vi "Analyse Doppler waveforms.vi"() -> ()   [LabVIEW 2022 SP3]
uses:
  Instance           1 33Saved   Analyse Doppler waveforms .vi
  Instance           6 33Saved   Analyse Doppler waveforms .vi
  Instance           5 33Saved   Analyse Doppler waveforms .vi
  Instance           2 33Saved   Analyse Doppler waveforms .vi
  <vilib>/express/express analysis/Spectral/Block/exnSpectralBlock spectral measurements power poly.vi
  <vilib>/express/express analysis/Spectral/Block/exnSpectralBlock spectral measurements power DDT.vi
  Instance           7 33Saved   Analyse Doppler waveforms .vi
  Instance           8 33Saved   Analyse Doppler waveforms .vi
  <vilib>/express/express analysis/Spectral/XNode/ExpressSpectralMeasurementsBlockNode.xnode
  <vilib>/gmath/NI_Gmath.lvlib
panel:
  out "Number of samples 2":dbl
  out "Waveform Graph 4":dbl[](graph)
  out "Array 3":dbl[](array[numeric])
  out "Array 2":i32[](array[numeric])
  out "cursor y  index":dbl
  out "cursor x  index":dbl
  out "Spectrogram":dbl[][](graph)
  out "Number of samples":i32
  in  "Frame time shift":i32(slide)=290 caption="in mumber of samples" min=4 max=512 step=2 scale=0.0..512.0
  out "Sampling frequency":dbl
  in  "window selector":i32(ring)=4 items=["Rectangular", "Blackman", "Hamming", "Hanning", "Gaussian"]
  out "Waveform Graph 3":dynamicdata(graph)=[{"t0"=timestamp(0 s since 1904-01-01), "dt"=31.372549019607842, "Y"=array[255 elements], "attributes"=variant("NI_ChannelName"=variant(string "Dev1/ai0 (Power Spectrum)"), "NI_ExpIsRelativeTime"=variant(bool TRUE), "NI_ExpStartTimeStamp"=variant(timestamp timestamp(3271175312.342312 s since 1904-01-01)), "NI_ExpTimeStamp"=variant(timestamp timestamp(3271175312.8210626 s since 1904-01-01)), "NI_ExpXDimension"=variant(string "f"), "NI_OriginalChannelName"=variant(string "Dev1/ai0"))}]
  in  "Frame width":i32(slide)=342 min=2 max=1024 step=2 scale=0.0..1024.0
  in  "stop":bool
  in  "Begin Sample":i32(slide)=2401 min=1 max=50000 step=10 scale=0.0..50000.0
  out "Waveform Graph 2":dynamicdata(graph)=[{"t0"=timestamp(0.15006250000000002 s since 1904-01-01), "dt"=6.25e-05, "Y"=array[510 elements], "attributes"=variant("NI_ChannelName"=variant(string "Dev1/ai0 (Extracted)"), "NI_ExpIsRelativeTime"=variant(bool TRUE), "NI_ExpStartTimeStamp"=variant(timestamp timestamp(3271175312.342312 s since 1904-01-01)), "NI_ExpTimeStamp"=variant(timestamp timestamp(3271175312.8210626 s since 1904-01-01)), "NI_ExpXDimension"=variant(string "t"), "NI_OriginalChannelName"=variant(string "Dev1/ai0"))}]
  out "Waveform Graph":dynamicdata(graph)=[{"t0"=timestamp(0 s since 1904-01-01), "dt"=6.25e-05, "Y"=array[5000 elements], "attributes"=variant("NI_ChannelName"=variant(string "Dev1/ai0"), "NI_ExpIsRelativeTime"=variant(bool TRUE), "NI_ExpStartTimeStamp"=variant(timestamp timestamp(3271175312.342312 s since 1904-01-01)), "NI_ExpTimeStamp"=variant(timestamp timestamp(3271175312.671 s since 1904-01-01)), "NI_ExpXDimension"=variant(string "t"))}]
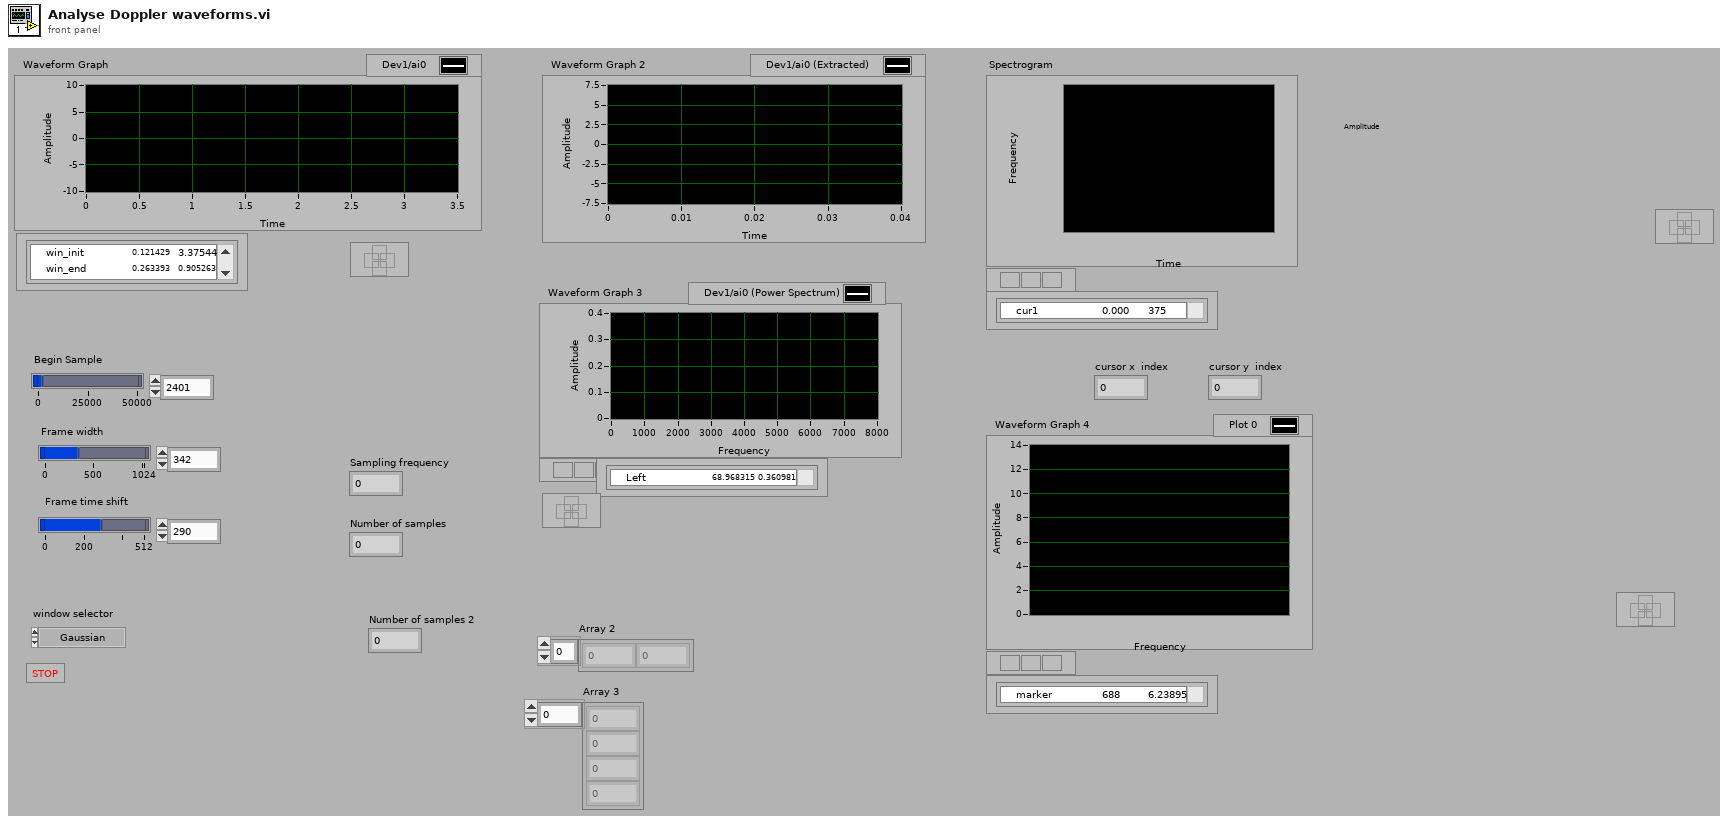
[diagram p1: front panel]
types:
  T1 = cluster{"averaging mode":u16, "weighting mode":u16, "number of averages":u32}
  T2 = cluster{"dB On (F)":bool, "unwrap phase (F)":bool, "convert to degree (F)":bool}
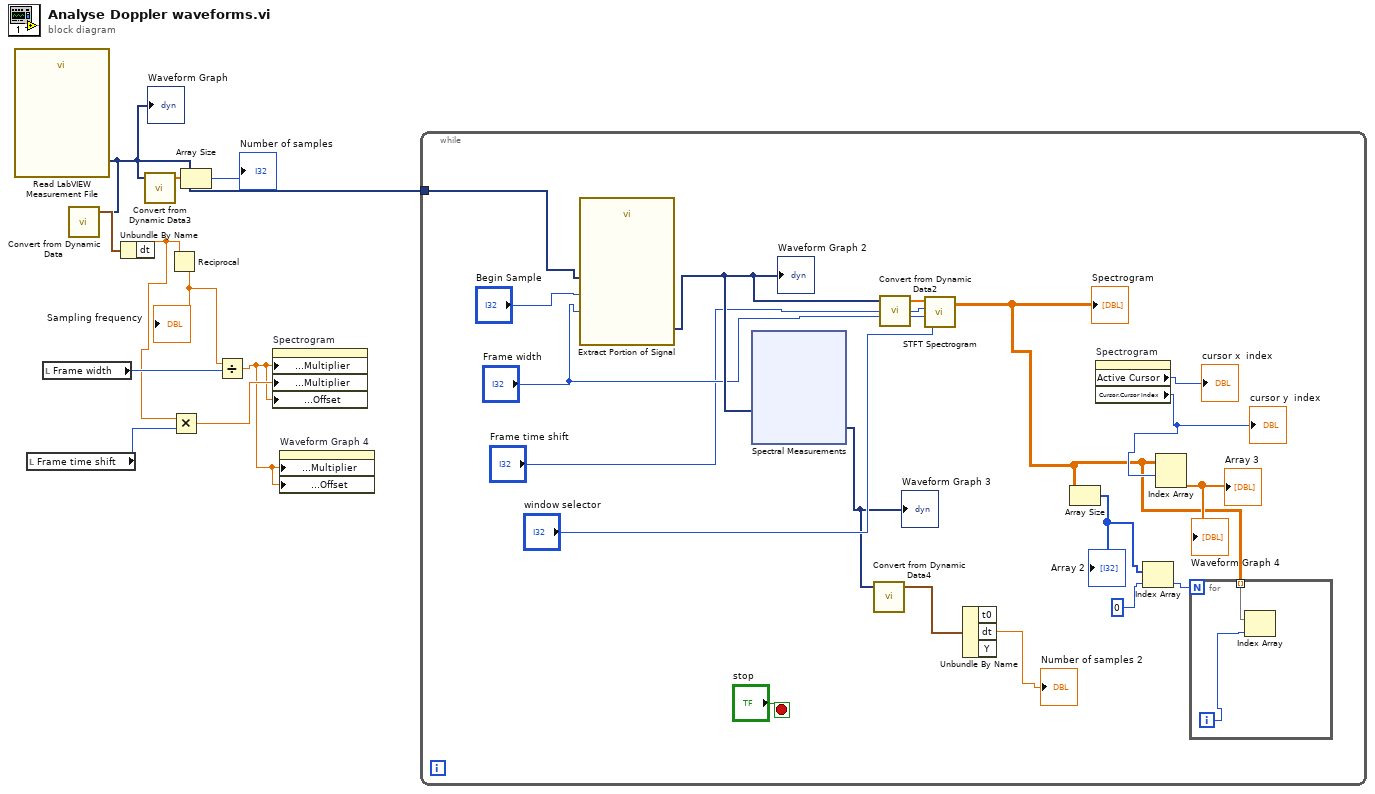
[diagram p0: block diagram]
diagram:
  n1 = call "Read LabVIEW Measurement File"() -> ("Signals"=w9:dynamicdata)  [unwired: 3 in, 8 out]
  "Waveform Graph" <- w9
  n2 = local read "Frame time shift"() -> (w4:i32)
  n3 = local read "Frame width"() -> (w5:i32)
  n4 = call "Convert from Dynamic Data"("Dynamic Data Type"=w9) -> ("Waveform"=w10:waveform(dbl))  [unwired: 1 in, 2 out]
  n5 = Unbundle By Name(w10) -> ("dt"=w3:dbl)
  n6 = call "Convert from Dynamic Data3"("Dynamic Data Type"=w9) -> ("Array"=w8:dbl[])  [unwired: 3 out]
  n7 = Reciprocal(x=w3) -> (1/x=w7:dbl)
  "Sampling frequency" <- w7
  n8 = Multiply(x=w3, y=w4) -> (x*y=w2:dbl)
  n9 = Array Size(array=w8) -> (size(s)=→"Number of samples":i32)
  n10 = Divide(x=w7, y=w5) -> (x/y=w1:dbl)
  n11 = property on="Spectrogram" class="IntGraph (strict)"("Y Scale.Offset and Multiplier:Multiplier"=w1, "X Scale.Offset and Multiplier:Multiplier"=w2, "Y Scale.Offset and Multiplier:Offset"=w1) -> ()  [unwired: 2 in, 2 out]
  n12 = property on="Waveform Graph 4" class="WFGraph (strict)"("X Scale.Offset and Multiplier:Multiplier"=w1, "X Scale.Offset and Multiplier:Offset"=w1) -> ()  [unwired: 2 in, 2 out]
  n13 = while {
    tunnel: w9 -> [w23]
    stop <- "stop" stop-if-true
    n14 = call "Extract Portion of Signal"("Samples"="Frame width", "Begin Sample"="Begin Sample", "Signals"=w23) -> ("Section"=w26:dynamicdata)  [unwired: 1 in, 7 out]
    "Waveform Graph 2" <- w26
    n15 = xnode "Spectral Measurements"("Signals"=w26) -> ("Power Spectrum"=w17:dynamicdata)  [unwired: 1 in, 1 out]
    "Waveform Graph 3" <- w17
    n16 = call "Convert from Dynamic Data4"("Dynamic Data Type"=w17) -> ("Waveform"=w16:waveform(dbl))  [unwired: 1 in, 2 out]
    n17 = call "Convert from Dynamic Data2"("Dynamic Data Type"=w26) -> ("Array"=w21:dbl[])  [unwired: 3 out]
    n18 = call <vilib>:"STFT Spectrogram.vi"("window selector"="window selector", "window length"="Frame width", "time increment"="Frame time shift", "X"=w21) -> ("STFT Spectrogram {X}"=w11:dbl[][])  [unwired: 1 out]
    "Spectrogram" <- w11
    n19 = Unbundle By Name(w16) -> ("dt"=→"Number of samples 2":dbl)  [unwired: 2 out]
    n20 = Array Size(array=w11) -> (size(s)=w14:i32[])
    "Array 2" <- w14
    n21 = property on="Spectrogram" class="IntGraph (strict)"() -> ("Active Cursor"=→"cursor x  index":u32, "Cursor.Cursor Index"=w19:i32)  [unwired: 2 in, 2 out]
    "cursor y  index" <- w19
    n22 = Index Array(array=w14, index=0) -> (element=w12:i32)
    n23 = Index Array(array=w11, index (row)=w19) -> (element=→"Array 3" →"Waveform Graph 4":dbl[])  [unwired: 1 in]
    n24 = for {
      N: w12 -> [_]
      tunnel: w11 -> [w39] mode=indexing
      i -> [w38]
      n25 = Index Array(array=w39, index=w38) -> ()  [unwired: 1 out]
    }
  }
